vi "Flatten Lines.vi"(8 "error in (no error)":errorcluster, 10 "Valid Point Indexes (flattened)":refnum<class "1D Array u32.lvclass">, 11 "Lines In":refnum<class "2D Array f32.lvclass">) -> (0 "error out":errorcluster, 3 "Flattened Lines Out":refnum<class "1D Array f32.lvclass">)   [LabVIEW 2020, in "G2CPU Line Profile.lvlib"]
uses:
  G2CPU Line Profile.lvlib
  <vilib>/Natan Biesmans/G2CPU GPU and CPU HPC Toolkit/G2CPU Libraries/Arrays/1DArray/f32/1D Array f32.lvclass
  C:/Program Files/National Instruments/LabVIEW 2025/vi.lib/Natan Biesmans/G2CPU GPU and CPU HPC Toolkit/G2CPU Libraries/Arrays/Array/Array Prototype.lvclass
  <vilib>/Natan Biesmans/G2CPU GPU and CPU HPC Toolkit/G2CPU Libraries/Arrays/1DArray/u32/1D Array u32.lvclass
  <vilib>/Natan Biesmans/G2CPU GPU and CPU HPC Toolkit/G2CPU Libraries/Arrays/2DArray/f32/2D Array f32.lvclass
  <vilib>/Natan Biesmans/G2CPU GPU and CPU HPC Toolkit/G2CPU Libraries/Arrays/Array/Array Prototype.lvclass/Array Prototype.ctl
  ad121926-9750-40df-aada-7dce03c98198.vi
  9936f39b-35c7-4ad4-a86e-a5a877eae4b3.vi
  91be072a-a482-4f8f-99c5-5d08104f7c0c.vi
  <vilib>/Natan Biesmans/G2CPU GPU and CPU HPC Toolkit/G2CPU Libraries/Arrays/Array/G2CPU Get Array Pointer.vi
  ad121926-9750-40df-aada-7dce03c98198.vi/e9bebd79-1c27-4fc1-b91f-30516104c7f0.vi
  9936f39b-35c7-4ad4-a86e-a5a877eae4b3.vi/7467a0f1-0650-4e63-b635-b3d2b2ec9a4e.vi
  9936f39b-35c7-4ad4-a86e-a5a877eae4b3.vi/8ee11bc3-5ef5-497e-97f0-8db2b3aaa149.vi
  9936f39b-35c7-4ad4-a86e-a5a877eae4b3.vi/c7af9698-5e3c-4e11-95da-3024075b67d2.vi
  91be072a-a482-4f8f-99c5-5d08104f7c0c.vi/2e03f477-51b7-4ba0-bb4f-4f838f6557e6.vi
  91be072a-a482-4f8f-99c5-5d08104f7c0c.vi/125d45d4-836b-469d-8a4a-6adb452f866d.vi
  91be072a-a482-4f8f-99c5-5d08104f7c0c.vi/8038e9ed-2e71-4568-91ba-0d873494c5ed.vi
  91be072a-a482-4f8f-99c5-5d08104f7c0c.vi/2e03f477-51b7-4ba0-bb4f-4f838f6557e6.vi/d8e2d9cc-c923-495e-b121-b6b84788c73f.vi
  91be072a-a482-4f8f-99c5-5d08104f7c0c.vi/2e03f477-51b7-4ba0-bb4f-4f838f6557e6.vi/345e91f0-9a5e-4de4-af9c-133346717e4a.vi
  <vilib>/Natan Biesmans/G2CPU GPU and CPU HPC Toolkit/G2CPU Libraries/Arrays/1DArray/s32/1D Array s32.lvclass
  <vilib>/Natan Biesmans/G2CPU GPU and CPU HPC Toolkit/ArrayFire Driver/VIs/transpose.vi
  <vilib>/Natan Biesmans/G2CPU GPU and CPU HPC Toolkit/G2CPU Libraries/Arrays/Array/G2CPU Release Array.vi
  <vilib>/Natan Biesmans/G2CPU GPU and CPU HPC Toolkit/G2CPU Libraries/Arrays/Array/G2CPU Set Array Pointer.vi
  <vilib>/Natan Biesmans/G2CPU GPU and CPU HPC Toolkit/ArrayFire Driver/VIs/flat.vi
  <vilib>/Natan Biesmans/G2CPU GPU and CPU HPC Toolkit/ArrayFire Driver/VIs/cast.vi
  <vilib>/Natan Biesmans/G2CPU GPU and CPU HPC Toolkit/ArrayFire Driver/VIs/lookup.vi
  <vilib>/Natan Biesmans/G2CPU GPU and CPU HPC Toolkit/G2CPU Libraries/Arrays/Array/Array Prototype.lvclass
  <vilib>/Natan Biesmans/G2CPU GPU and CPU HPC Toolkit/G2CPU Libraries/Arrays/DataTypes/f32/f32.lvclass
  <vilib>/Natan Biesmans/G2CPU GPU and CPU HPC Toolkit/G2CPU Libraries/Arrays/2DArray/2D Array Prototype.lvclass
  <vilib>/Natan Biesmans/G2CPU GPU and CPU HPC Toolkit/G2CPU Libraries/Arrays/DataTypes/I32/s32.lvclass
  <vilib>/Natan Biesmans/G2CPU GPU and CPU HPC Toolkit/G2CPU Libraries/Arrays/1DArray/1D Array Prototype.lvclass
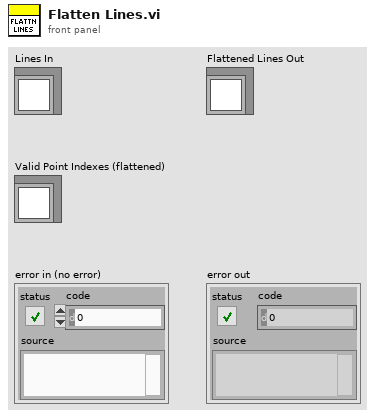
[diagram p1: front panel]
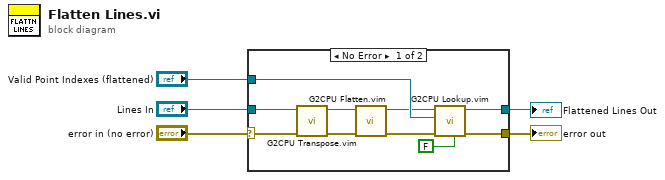
[diagram p0: block diagram]
diagram:
  n1 = case shown="No Error" "error in (no error)" {
    selector: "error in (no error)" -> [w15 _]
    tunnel: [w12 _] -> w4
    tunnel: "Valid Point Indexes (flattened)" -> [w11 _]
    tunnel: [w10 _] -> w2
    tunnel: "Lines In" -> [w7 _]
    frame No Error {
      n2 = call "G2CPU Transpose.vim"("error in (no error)"=w15, "Array In"=w7) -> ("error out"=w14:errorcluster, "Array out"=w6:refnum<class "2D Array f32.lvclass">)  [unwired: 8 in]
      n3 = call "G2CPU Flatten.vim"("error in (no error)"=w14, "Array In"=w6) -> ("error out"=w13:errorcluster, "Array out"=w8:refnum<class "1D Array f32.lvclass">)  [unwired: 8 in]
      n4 = call "G2CPU Lookup.vim"("Auto Release Indices (Enabled)"=FALSE, "error in (no error)"=w13, "Indices (1D)"=w11, "Array In"=w8) -> ("error out"=w10:errorcluster, "Indexed Array"=w12:refnum<class "1D Array f32.lvclass">)  [unwired: 6 in]
    }
    frame Error {
    }
  }
  "Flattened Lines Out" <- w4
  "error out" <- w2
